vi "TurretChooseAngle.vi"(3 "Zero Turret":bool, 4 "Goal Angle (deg)":dbl format="%#_13g", 5 "Current Angle (deg)":dbl format="%#_13g") -> (0 "In Deadzone":bool, 1 "Angular Distance (deg)":dbl format="%_4g")   [LabVIEW 2019]
panel:
  in  "Deadzone Max(deg)":dbl=94.0 format="%#_13g"
  in  "Deadzone Min(deg)":dbl=87.0 format="%#_13g"
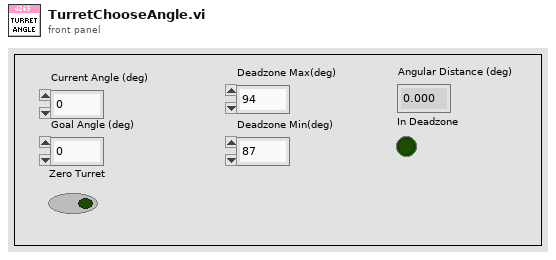
[diagram p1: front panel]
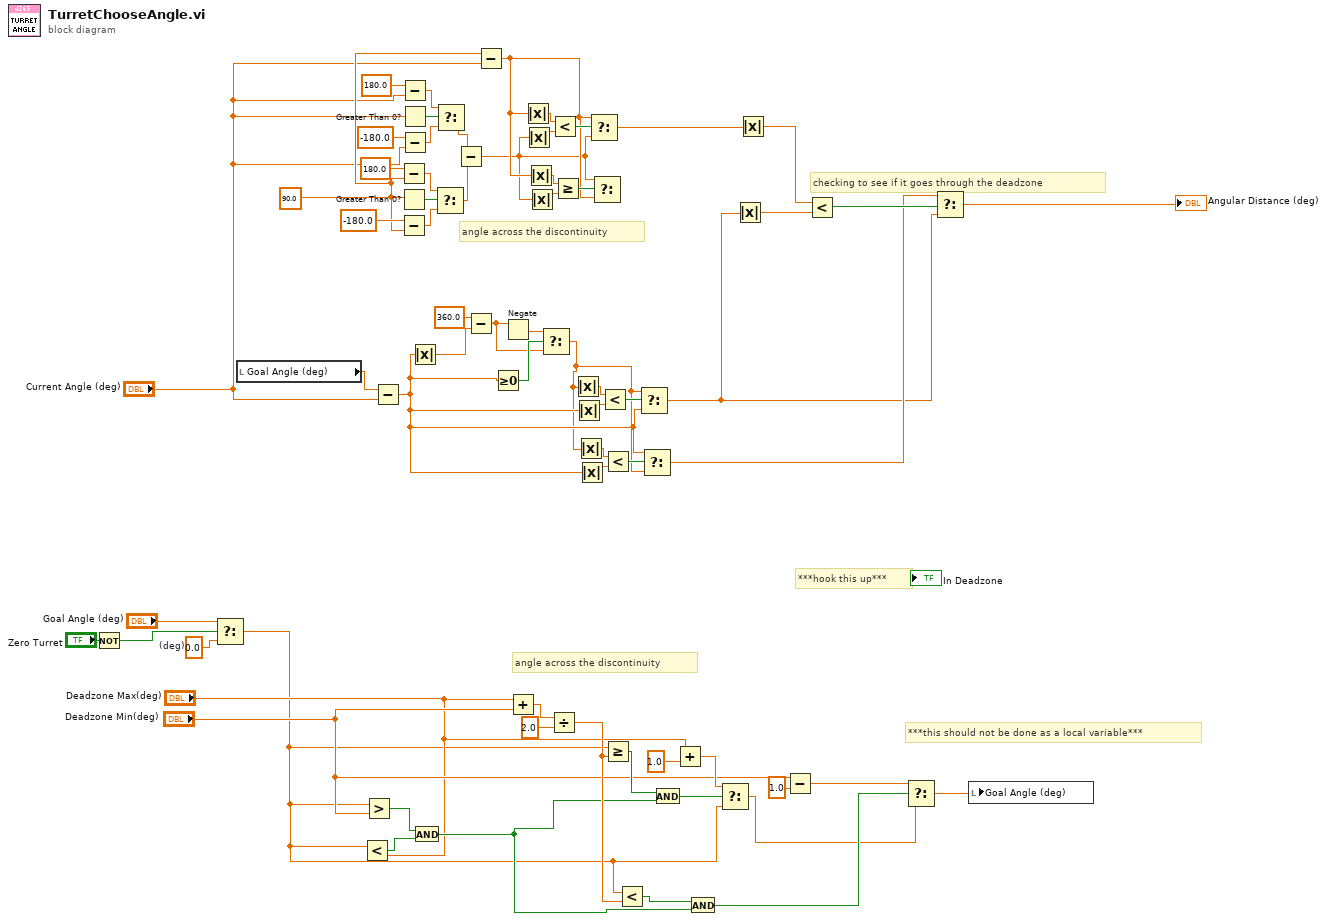
[diagram p0: block diagram]
diagram:
  w18 = 90.0 ("y")
  w61 = 0.0  # (deg)
  # "***hook this up***"
  # "***this should not be done as a local variable***"
  # "checking to see if it goes through the deadzone"
  # "angle across the discontinuity"
  # "angle across the discontinuity"
  n1 = Not(x="Zero Turret") -> (.not. x?=w62:bool)
  n2 = Select(t="Goal Angle (deg)", s=w62, f=w61) -> (s? t:f=w16:dbl)
  n3 = local read "Goal Angle (deg)"() -> (w3:dbl)
  n4 = Less?(x=w16, y="Deadzone Max(deg)") -> (x < y?=w54:bool)
  n5 = Greater?(x=w16, y="Deadzone Min(deg)") -> (0:w53:bool)
  n6 = Subtract(x=w3, y="Current Angle (deg)") -> (x-y=w7:dbl)
  n7 = Subtract(x=180.0, y=w18) -> (x-y=w31:dbl)
  n8 = Greater Than 0?(x=w18) -> (x > 0?=w33:bool)
  n9 = Subtract(x=-180.0, y=w18) -> (x-y=w29:dbl)
  n10 = Subtract(x=180.0, y="Current Angle (deg)") -> (x-y=w28:dbl)
  n11 = Greater Than 0?(x="Current Angle (deg)") -> (x > 0?=w36:bool)
  n12 = Subtract(x=-180.0, y="Current Angle (deg)") -> (x-y=w27:dbl)
  n13 = Absolute Value(x=w7) -> (abs(x)=w1:dbl)
  n14 = And(x=w53, y=w54) -> (x .and. y?=w46:bool)
  n15 = Select(t=w31, s=w33, f=w29) -> (s? t:f=w26:dbl)
  n16 = Select(t=w28, s=w36, f=w27) -> (s? t:f=w25:dbl)
  n17 = Subtract(x=w25, y=w26) -> (x-y=w19:dbl)
  n18 = Subtract(x=360.0, y=w1) -> (x-y=w5:dbl)
  n19 = Subtract(x=w18, y="Current Angle (deg)") -> (x-y=w20:dbl)
  n20 = Greater Or Equal To 0?(x=w7) -> (x >= 0?=w8:bool)
  n21 = Negate(x=w5) -> (-x=w6:dbl)
  n22 = Add(x="Deadzone Max(deg)", y="Deadzone Min(deg)") -> (x+y=w56:dbl)
  n23 = Absolute Value(x=w20) -> (abs(x)=w37:dbl)
  n24 = Absolute Value(x=w19) -> (abs(x)=w38:dbl)
  n25 = Absolute Value(x=w20) -> (abs(x)=w22:dbl)
  n26 = Absolute Value(x=w19) -> (abs(x)=w23:dbl)
  n27 = Select(t=w6, s=w8, f=w5) -> (s? t:f=w4:dbl)
  n28 = Divide(x=w56, y=2.0) -> (x/y=w48:dbl)
  n29 = Less?(x=w37, y=w38) -> (x < y?=w24:bool)
  n30 = Greater Or Equal?(x=w22, y=w23) -> (x >= y?=w21:bool)
  n31 = Absolute Value(x=w4) -> (abs(x)=w65:dbl)
  n32 = Absolute Value(x=w7) -> (abs(x)=w66:dbl)
  n33 = Absolute Value(x=w4) -> (abs(x)=w58:dbl)
  n34 = Absolute Value(x=w7) -> (abs(x)=w59:dbl)
  n35 = Select(t=w20, s=w24, f=w19) -> (s? t:f=w12:dbl)
  n36 = Select(t=w19, s=w21, f=w20) -> ()  [unwired: 1 out]
  n37 = Less?(x=w65, y=w66) -> (x < y?=w60:bool)
  n38 = Less?(x=w58, y=w59) -> (x < y?=w57:bool)
  n39 = Greater Or Equal?(x=w16, y=w48) -> (x >= y?=w52:bool)
  n40 = Less?(x=w16, y=w48) -> (x < y?=w47:bool)
  n41 = Select(t=w4, s=w60, f=w7) -> (s? t:f=w14:dbl)
  n42 = Select(t=w7, s=w57, f=w4) -> (s? t:f=w15:dbl)
  n43 = And(x=w52, y=w46) -> (x .and. y?=w51:bool)
  n44 = Add(x="Deadzone Max(deg)", y=1.0) -> (x+y=w49:dbl)
  n45 = And(x=w47, y=w46) -> (x .and. y?=w45:bool)
  n46 = Select(t=w49, s=w51, f=w16) -> (s? t:f=w42:dbl)
  n47 = Absolute Value(x=w14) -> (abs(x)=w10:dbl)
  n48 = Absolute Value(x=w12) -> (abs(x)=w11:dbl)
  n49 = Subtract(x="Deadzone Min(deg)", y=1.0) -> (x-y=w43:dbl)
  n50 = Less?(x=w11, y=w10) -> (x < y?=w17:bool)
  n51 = Select(t=w43, s=w45, f=w42) -> (s? t:f=w41:dbl)
  n52 = Select(t=w15, s=w17, f=w14) -> (s? t:f=→"Angular Distance (deg)":dbl)
  n53 = local write "Goal Angle (deg)"(w41) -> ()
